vi "Initialize Transfer Groups.vi"(8 "error in (no error)":errorcluster, 10 "Group Configurations":refnum<class "Group Configuration.lvclass">[](array[class]), 11 "UDP Transceiver in":refnum<class "UDP Transceiver.lvclass">) -> (0 "error out":errorcluster, 3 "UDP Transceiver out":refnum<class "UDP Transceiver.lvclass">)   [LabVIEW 2017, in "DSF Core.lvlib" / "UDP Transceiver.lvclass"]
uses:
  UDP Transceiver.lvclass
  Transfer Parameters.ctl
  Transfer Group Parameters.ctl
  Classes/Configuration Session/Configuration Session.lvclass
  Throw Unknown Setting Error.vi
  Classes/Configuration/Runtime/Runtime Configuration.lvclass
  Classes/Configuration/Base/Group/Group Configuration.lvclass
  C:/Git/DSF/Core/Classes/Configuration/Runtime/Runtime Configuration.lvclass
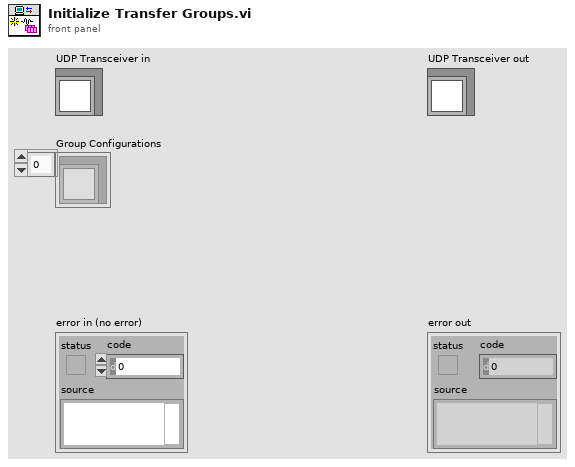
[diagram p1: front panel]
types:
  T1 = typedef "DSF Core.lvlib/UDP Transceiver.lvclass/Transfer Group Parameters.ctl" = cluster{"transfers":T2[], "max size":i32, "timeout":i32}
  T2 = typedef "DSF Core.lvlib/UDP Transceiver.lvclass/Transfer Parameters.ctl" = cluster{"group offset":u64, "size":u64, "address":u32, "port":u16}
  T3 = typedef "DSF Core.lvlib/DSF Settings Info.ctl" = cluster{"component":string, "version":T4, "values":cluster{"key":string, "value":string}[]}
  T4 = typedef "DSF Core.lvlib/DSF Version Info.ctl" = cluster{"major":u32, "minor":u32, "fix":u32, "build":string}
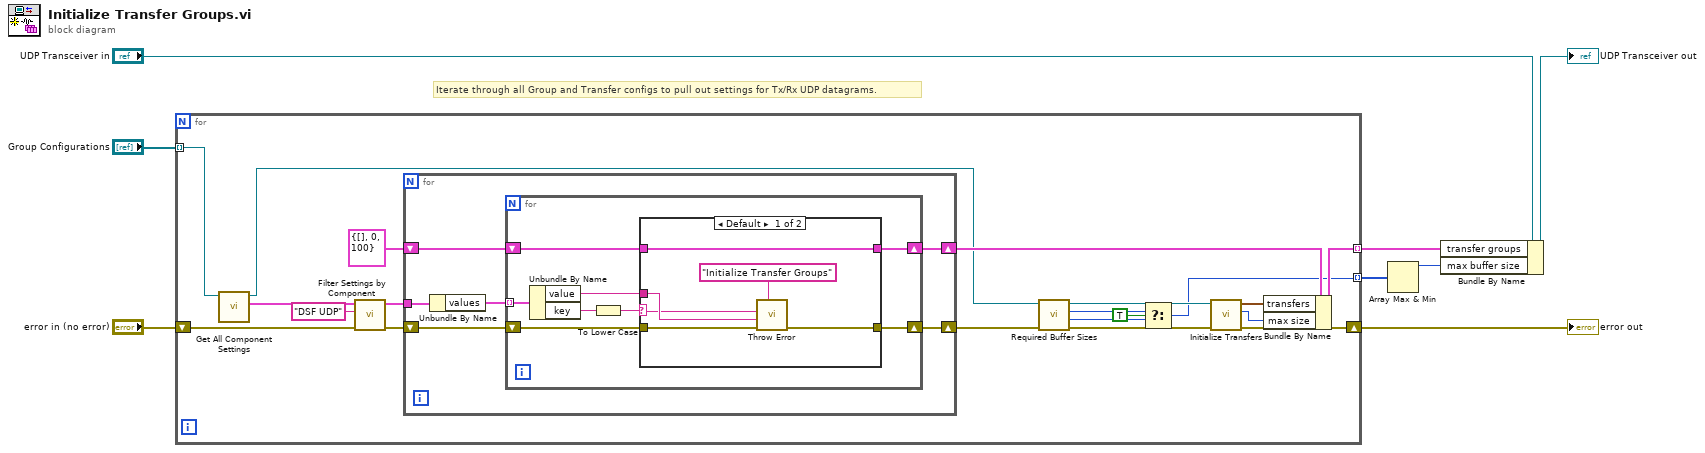
[diagram p0: block diagram]
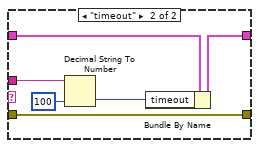
[diagram p2: hidden frame]
diagram:
  # "Iterate through all Group and Transfer configs to pull out settings for Tx/Rx UDP datagrams."
  n1 = for {
    tunnel: "Group Configurations" -> [w11] mode=indexing
    shift-right: [w28] -> w7
    shift-left: "error in (no error)" -> [w15]
    tunnel: [w18] -> w5 mode=indexing
    tunnel: [w24] -> w4 mode=indexing
    n2 = call "Get All Component Settings.vi"("Runtime Configuration in"=w11) -> ("component settings"=w12:T3, "Runtime Configuration out"=w10:refnum<class "Group Configuration.lvclass">)  [unwired: 8 in, 1 out]
    n3 = call "Filter Settings by Component.vi"("error in (no error)"=w15, "component"="DSF UDP", "settings"=w12) -> ("error out"=w14:errorcluster, "filtered settings"=w13:T3)  [unwired: 7 in]
    n4 = for {
      tunnel: w13 -> [w30]
      shift-right: [w32] -> w25
      shift-left: T1 {"transfers"=[], "max size"=0, "timeout"=100} ("Rx/Tx Parameters") -> [w33]
      shift-right: [w34] -> w22
      shift-left: w14 -> [w31]
      n5 = Unbundle By Name(w30) -> ("values"=w29:cluster{"key":string, "value":string}[])
      n6 = for {
        tunnel: w29 -> [w39] mode=indexing
        shift-right: [w40] -> w34
        shift-left: w31 -> [w41]
        shift-right: [w38] -> w32
        shift-left: w33 -> [w37]
        n7 = Unbundle By Name(w39) -> ("value"=w36:string, "key"=w42:string)
        n8 = To Lower Case(string=w42) -> (all lower case string=w35:string)
        n9 = case shown="Default" w35 {
          selector: w35 -> [w43 _]
          tunnel: w36 -> [w46 w54]
          tunnel: w41 -> [w45 w51]
          tunnel: [w44 w51] -> w40
          tunnel: w37 -> [w47 w49]
          tunnel: [w47 w50] -> w38
          frame Default {
            n10 = call-poly "Throw Error.vi"("source vi name"="Initialize Transfer Groups", "error in (no error)"=w45, "value"=w46, "key"=w43) -> ("error out"=w44:errorcluster)  [unwired: 7 in]
          }
          frame "timeout" {
            n11 = Decimal String To Number(string=w54, default (0L)=100 ("default (0 I32)")) -> (number=w52:i32)  [unwired: 1 in, 1 out]
            n12 = Bundle By Name(cluster=w49, "timeout"=w52) -> (w50:T1)
          }
        }
      }
    }
    n13 = call-dynamic "Required Buffer Sizes.vi"("error in (no error)"=w22, "Group Configuration in"=w10) -> ("error out"=w21:errorcluster, "string size"=w20:u64, "engine size"=w23:u64, "Group Configuration out"=w19:refnum<class "Group Configuration.lvclass">)  [unwired: 6 in]
    n14 = Select(t=w23, s=TRUE, f=w20) -> (s? t:f=w18:u64)
    n15 = call "Initialize Transfers.vi"("error in (no error)"=w21, "Group Configuration"=w19) -> ("error out"=w28:errorcluster, "max buffer size"=w17:u64, "transfer parameters"=w26:T2[])  [unwired: 7 in]
    n16 = Bundle By Name(cluster=w25, "transfers"=w26, "max size"=w17) -> (w24:T1)
  }
  "error out" <- w7
  n17 = Array Max & Min(array=w5) -> (max value=w1:u64)  [unwired: 3 out]
  n18 = Bundle By Name(cluster="UDP Transceiver in", "transfer groups"=w4, "max buffer size"=w1) -> (→"UDP Transceiver out":refnum<class "UDP Transceiver.lvclass">)
